vi "HeaderAction.vi"(0 "InstrClass":refnum<class "Monospec50.lvclass"> caption="DNL_LabVIEW Object in", 11 "error in (no error)":errorcluster caption="entrée d'erreur (pas d'erreur)") -> (4 "InstrClassOut":refnum<class "Monospec50.lvclass"> caption="DNL_LabVIEW Object out", 6 "DataNames":string[](array[string]), 8 "Instr Name":string, 10 "HeaderString":string, 13 "ArrDisplayNames":string[](array[string]), 14 "DisplayNames":string[](array[string]), 15 "error out":errorcluster caption="sortie d'erreur")   [LabVIEW 2019, in "Monospec50.lvclass"]
uses:
  Monospec50.lvclass
  C:/Programmes Labview/LabScanV1A/DevicesClass/BaseDevice/BaseDevice.lvclass
  Monospec50.lvclass/Monospec50.ctl
  BaseDevice/BaseDevice.lvclass
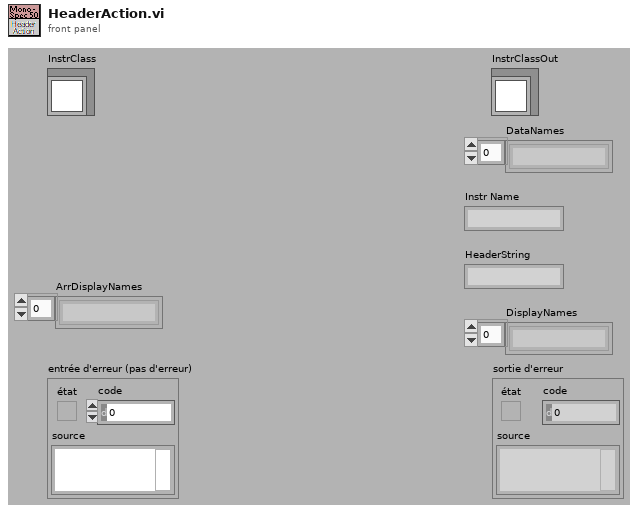
[diagram p1: front panel]
types:
  T1 = typedef "Monospec50.lvclass/Monospec50_Func.ctl" = enum16{"Position (nm)"}
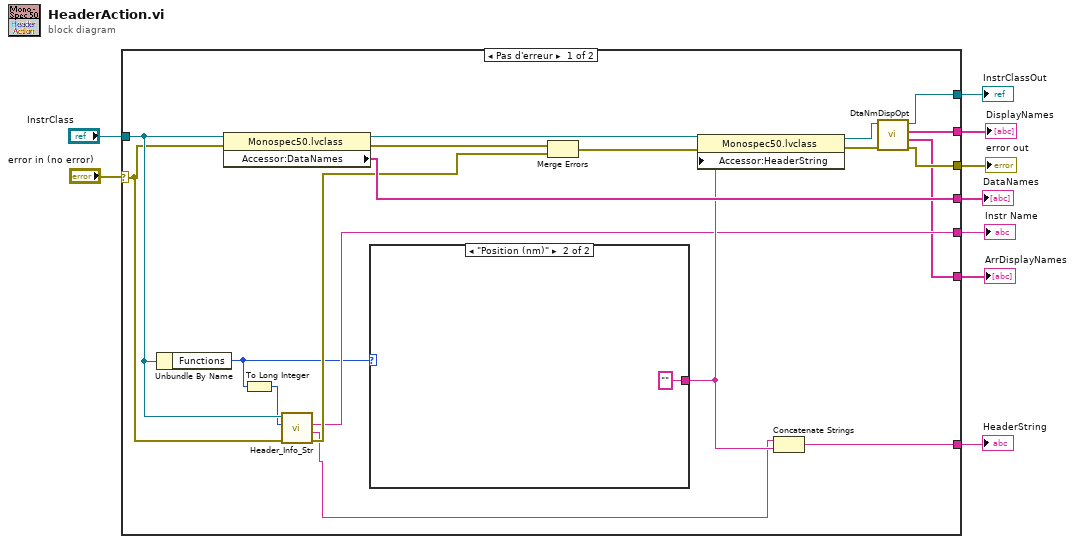
[diagram p0: block diagram]
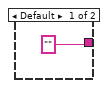
[diagram p2: hidden frame]
diagram:
  n1 = case shown="Pas d'erreur" "error in (no error)" {
    selector: "error in (no error)" -> [w16 w31]
    tunnel: [w19 _] -> w8
    tunnel: [w28 _] -> w7
    tunnel: "InstrClass" -> [w17 w32]
    tunnel: [w23 w31] -> w5
    tunnel: [w22 w32] -> w3
    tunnel: [w13 _] -> w4
    tunnel: [w20 _] -> w2
    tunnel: [w10 _] -> w1
    frame No Error {
      n2 = Unbundle By Name(w17) -> ("Functions"=w12:T1)
      n3 = property class="Monospec50.lvclass"(reference=w17, error in=w16) -> (reference out=w27:refnum<class "Monospec50.lvclass">, error out=w26:errorcluster, "Accessor:DataNames"=w28:string[])
      n4 = To Long Integer(number=w12) -> (32bit integer=w11:i32)
      n5 = call-dynamic "Header_Info_Str.vi"("error in (no error)"=w16, "Functions"=w11, "DefaultDev in"=w17) -> ("error out"=w15:errorcluster, "HdrInfoStr"=w14:string, "InstrumentName"=w13:string)  [unwired: 5 in, 1 out]
      n6 = case shown="\"Position (nm)\"" w12 {
        tunnel: ["" ("HeaderString") "" ("HeaderString")] -> w25
        frame Default {
        }
        frame "Position (nm)" {
        }
      }
      n7 = Merge Errors(w26, w15) -> (w18:errorcluster)
      n8 = property class="Monospec50.lvclass"(reference=w27, error in=w18, "Accessor:HeaderString"=w25) -> (reference out=w21:refnum<class "Monospec50.lvclass">, error out=w24:errorcluster)
      n9 = Concatenate Strings(w14, w25) -> (w19:string)
      n10 = call "DtaNmDispOpt.vi"("error in (no error)"=w24, "BaseDevice en entrée"=w21) -> ("error out"=w23:errorcluster, "ArrDisplayNames"=w10:string[], "DisplayNames"=w20:string[], "BaseDevice en sortie"=w22:refnum<class "Monospec50.lvclass">)  [unwired: 6 in]
    }
    frame Error {
    }
  }
  "error out" <- w5
  "InstrClassOut" <- w3
  "DataNames" <- w7
  "HeaderString" <- w8
  "Instr Name" <- w4
  "DisplayNames" <- w2
  "ArrDisplayNames" <- w1
